vi "Create Memory Cache.vi"(8 "error in (no error)":errorcluster, 10 "Transfers":refnum<class "Transfer.lvclass">[](array[class]), 11 "Transfers Groups":refnum<class "Transfer Group.lvclass">[](array[class])) -> (0 "error out":errorcluster, 3 "Cache out":refnum<class "Memory Cache.lvclass">)   [LabVIEW 2017, in "Data Sharing Framework Core.lvlib" / "Data Sharing Framework Engine.lvlib" / "Memory Cache.lvclass"]
uses:
  Memory Cache.lvclass
  Transfer/Transfer.lvclass
  Transfer Group/Transfer Group.lvclass
  Memory Cache.lvclass/Memory Cache.ctl
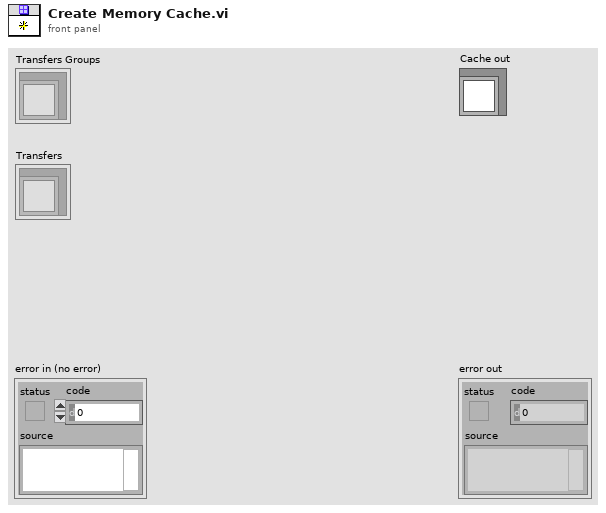
[diagram p1: front panel]
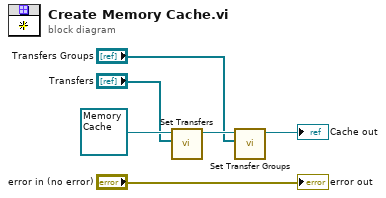
[diagram p0: block diagram]
diagram:
  n1 = call "Set Transfers.vi"("Transfers"="Transfers", "Cache in"=refnum<class "Memory Cache.lvclass"> refnum) -> ("Cache out"=w4:refnum<class "Memory Cache.lvclass">)  [unwired: 9 in]
  n2 = call "Set Transfer Groups.vi"("Transfers Groups"="Transfers Groups", "Cache in"=w4) -> ("Cache out"=→"Cache out":refnum<class "Memory Cache.lvclass">)  [unwired: 9 in]
  "error out" <- "error in (no error)"
